vi "write-to-mat-file-subvi.vi"(4 "Header2 file data":T5, 6 "Number of frames":u32, 7 "first frame number":u32, 8 "Error In":errorcluster, 9 "Header file data":T1 {"Pixel depth" items=["8 bits", "16 bits", "Float", "Complex", "RGB", "HSL"]}, 10 "Movie file name":string, 11 "Description Info":string) -> (0 "Error Out":errorcluster)   [LabVIEW 2014]
uses:
  ctt's/Header2 file.ctl
  ctt's/header1 file.ctl
  Glimpse-master/Glimpse core/Seq file v 1/Offset table.ctl
  Glimpse-master/Glimpse core/Seq file v 1/Offset.ctl
  Glimpse-master/Glimpse core/Seq file v 1/file number.ctl
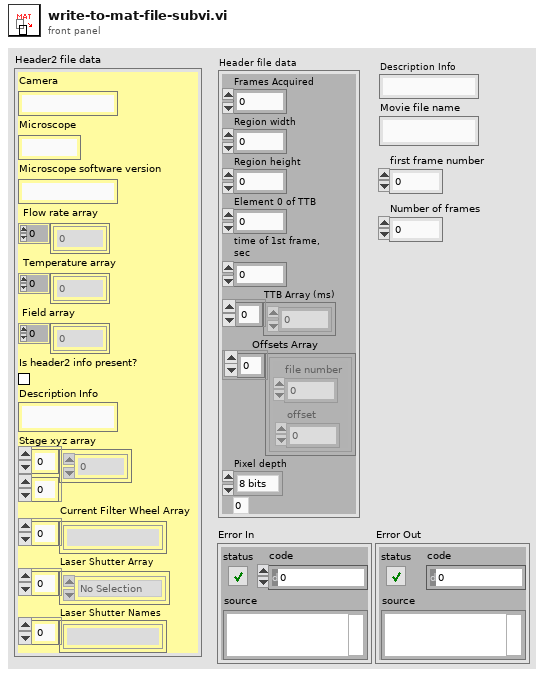
[diagram p1: front panel]
types:
  T1 = typedef "header1 file.ctl" = cluster{"Frames Acquired":u32, "Region width":i32, "Region height":i32, "Element 0 of TTB":u32, "time of 1st frame, \nsec":dbl, "TTB Array (ms)":u32[], "Offsets Array":T2, "Pixel depth":u32}
  T2 = typedef "Offset table.ctl" = cluster{"offset":T3, "file number":T4}[]
  T3 = typedef "Offset.ctl" = i32
  T4 = typedef "file number.ctl" = u8
  T5 = typedef "Header2 file.ctl" = cluster{"Camera":string, "Microscope":string, "Microscope software version":string, "Flow rate array":dbl[], "Temperature array":dbl[], "Field array":u16[], "Is header2 info present?":bool, "Description Info":string, "Stage xyz array":dbl[][], "Current Filter Wheel Array":string[], "Laser Shutter Array":enum32{"No Selection", "GFP", "Cy3 Long \nPass", "Cy3", "Cy5", "Off", "IR"}[], "Laser Shutter Names":string[]}
  T6 = enum32{"No Selection", "GFP", "Cy3 Long \nPass", "Cy3", "Cy5", "Off", "IR"}[]
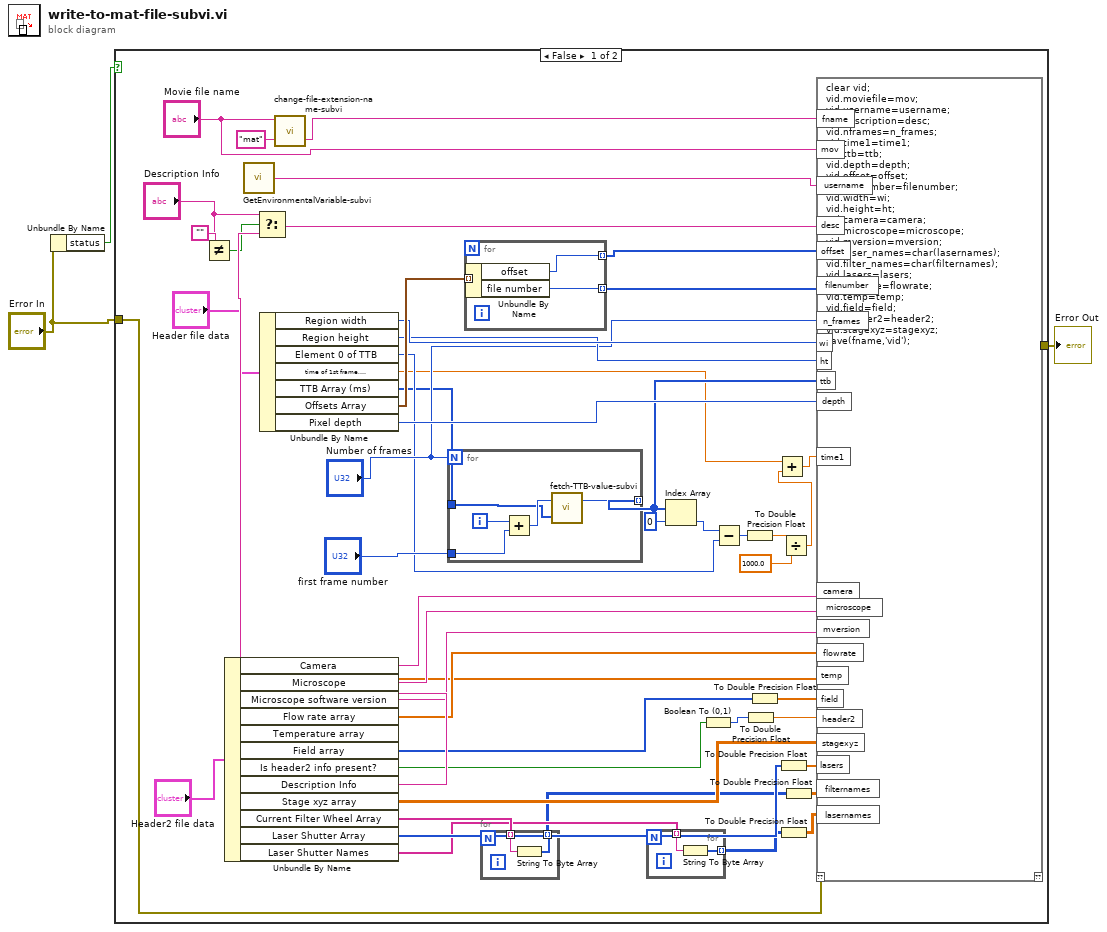
[diagram p0: block diagram]
diagram:
  n1 = Unbundle By Name("Error In") -> ("status"=w3:bool)
  n2 = case shown="False" w3 {
    tunnel: "Error In" -> [w25 w67]
    tunnel: [w33 w67] -> w1
    frame False {
      n3 = Not Equal?(x="Description Info", y="") -> (x != y?=w47:bool)
      n4 = Unbundle By Name("Header2 file data") -> ("Camera"=w44:string, "Microscope"=w43:string, "Microscope software version"=w42:string, "Flow rate array"=w32:dbl[], "Temperature array"=w31:dbl[], "Field array"=w30:u16[], "Is header2 info present?"=w28:bool, "Description Info"=w48:string, "Stage xyz array"=w26:dbl[][], "Current Filter Wheel Array"=w21:string[], "Laser Shutter Array"=w22:T6, "Laser Shutter Names"=w20:string[])
      n5 = call "GetEnvironmentalVariable-subvi.vi"() -> ("Value"=w51:string)  [unwired: 2 in]
      n6 = Select(t="Description Info", s=w47, f=w48) -> (s? t:f=w50:string)
      n7 = Unbundle By Name("Header file data") -> ("Region width"=w38:i32, "Region height"=w37:i32, "Element 0 of TTB"=w13:u32, "time of 1st frame, \nsec"=w6:dbl, "TTB Array (ms)"=w5:u32[], "Offsets Array"=w41:T2, "Pixel depth"=w36:u32)
      n8 = call "change-file-extension-name-subvi.vi"("New Extension (no period)"="mat", "Path String In"="Movie file name") -> ("New Path String Out"=w53:string)  [unwired: 1 out]
      n9 = for {
        N: "Number of frames" -> [_]
        tunnel: "first frame number" -> [w62]
        tunnel: [w60] -> w9 mode=indexing
        tunnel: w5 -> [w59]
        i -> [w63]
        n10 = Add(x=w63, y=w62) -> (x+y=w61:u32)
        n11 = call "fetch-TTB-value-subvi.vi"("Array of TTB Values (ms)"=w59, "Logical Frame Number\n(starting with zero)"=w61) -> ("TTB value out"=w60:u32)  [unwired: 1 out]
      }
      n12 = for {
        tunnel: w41 -> [w66] mode=indexing
        tunnel: [w65] -> w39 mode=indexing
        tunnel: [w64] -> w40 mode=indexing
        n13 = Unbundle By Name(w66) -> ("offset"=w65:T3, "file number"=w64:T4)
      }
      n14 = for {
        tunnel: w21 -> [w58] mode=indexing
        tunnel: [w57] -> w19 mode=indexing
        n15 = String To Byte Array(string=w58) -> (unsigned byte array=w57:u8[])
      }
      n16 = for {
        tunnel: w20 -> [w56] mode=indexing
        tunnel: [w55] -> w18 mode=indexing
        n17 = String To Byte Array(string=w56) -> (unsigned byte array=w55:u8[])
      }
      n18 = Index Array(array=w9, index=0) -> (element=w14:u32)
      n19 = Boolean To (0,1)(Boolean=w28) -> (0, 1=w29:i16)
      n20 = Subtract(x=w14, y=w13) -> (x-y=w12:u32)
      n21 = To Double Precision Float(number=w12) -> (double precision float=w11:dbl)
      n22 = To Double Precision Float(number=w29) -> (double precision float=w27:dbl)
      n23 = To Double Precision Float(number=w30) -> (double precision float=w24:dbl[])
      n24 = To Double Precision Float(number=w22) -> (double precision float=w23:dbl[])
      n25 = To Double Precision Float(number=w18) -> (double precision float=w17:dbl[][])
      n26 = Divide(x=w11, y=1000.0) -> (x/y=w7:dbl)
      n27 = Add(x=w6, y=w7) -> (x+y=w8:dbl)
      n28 = To Double Precision Float(number=w19) -> (double precision float=w16:dbl[][])
      n29 = script code="clear vid;\nvid.moviefile=mov;\nvid.username=username;\nvid.description=desc;\nvid.nframes=n_frames;\nvid.time1=time1;\nvid.ttb=ttb;\nvid.depth=depth;\nvid.offset=offset;\nvid.filenumber=filenumber;\nvid.width=wi;\nvid.height=ht;\nvid.camera=camera;\nvid.microscope=microscope;\nvid.mversion=mversion;\nvid.laser_names=char(lasernames);\nvid.filter_names=char(filternames);\nvid.lasers=lasers;\nvid.flowrate=flowrate;\nvid.temp=temp;\nvid.field=field;\nvid.header2=header2;\nvid.stagexyz=stagexyz;\nsave(fname,'vid');"("??"=w25, "fname"=w53, "mov"="Movie file name", "username"=w51, "desc"=w50, "filenumber"=w40, "n_frames"="Number of frames", "wi"=w38, "ht"=w37, "ttb"=w9, "depth"=w36, "time1"=w8, "camera"=w44, "microscope"=w43, "mversion"=w42, "offset"=w39, "flowrate"=w32, "temp"=w31, "field"=w24, "header2"=w27, "stagexyz"=w26, "lasers"=w23, "filternames"=w16, "lasernames"=w17) -> ("??"=w33:errorcluster)
    }
    frame True {
    }
  }
  "Error Out" <- w1
